vi "Read configuration.vi"(7 "force loading?":bool=TRUE, 8 "error in (no error)":errorcluster, 11 "Galvo in":refnum<class "ImagingModeSPIM.lvclass">) -> (0 "error out":errorcluster, 3 "Galvo out":refnum<class "ImagingModeSPIM.lvclass">)   [LabVIEW 2012, in "ImagingModeSPIM.lvclass"]
doc: "Reads the XML-based configuration file and populates the configuration cluster accordingly. Configuration file name is <component ID>.xml."
uses:
  ImagingModeSPIM.lvclass
  <vilib>/Distrio/Murmex/Murmex/Murmex.lvclass
  ImagingModeSPIM.lvclass/ImagingModeSPIM.ctl
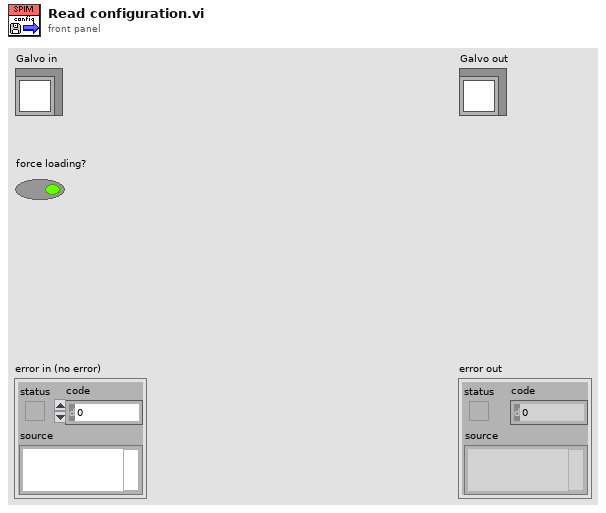
[diagram p1: front panel]
types:
  T1 = typedef "ImagingModeSPIM.lvclass/configuration_cluster.ctl" = cluster{"Sampling rate":dbl, "Samples per channel":i32, "Number of channels":T2, "Task cluster":T3}
  T2 = typedef "ImagingModeSPIM.lvclass/number of channels.ctl" = enum16{"empty", "double sided + PC", "double sided + WFS"}
  T3 = typedef "ImagingModeSPIM.lvclass/task_cluster.ctl" = cluster{"min Voltage":dbl[unit], "max Voltage":dbl[unit], "physical channel":string}
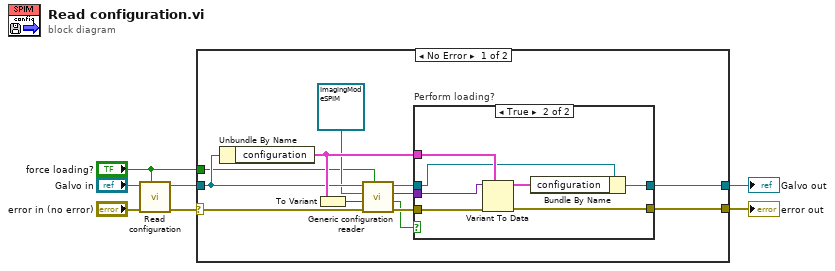
[diagram p0: block diagram]
diagram:
  n1 = call-parent "Read configuration.vi"("force loading?"="force loading?", "error in (no error)"="error in (no error)", "Murmex in"="Galvo in") -> ("error out"=w5:errorcluster, "Murmex out"=w4:refnum<class "ImagingModeSPIM.lvclass">)  [unwired: 7 in]
  n2 = case shown="No Error" w5 {
    selector: w5 -> [w15 w29]
    tunnel: w4 -> [w14 w30]
    tunnel: [w18 w29] -> w3
    tunnel: [w17 w30] -> w2
    tunnel: "force loading?" -> [w9 _]
    frame No Error {
      n3 = Unbundle By Name(w14) -> ("configuration"=w19:T1)
      n4 = To Variant(anything=w19) -> (Variant=w16:variant)
      n5 = call <vilib>:"Generic configuration reader.vi"("force loading?"=w9, "error in (no error)"=w15, "configuration cluster variant"=w16, "inheritance level"=refnum<class "ImagingModeSPIM.lvclass"> refnum ("Galvo.lvclass"), "Murmex in"=w14) -> ("error out"=w12:errorcluster, "loaded?"=w8:bool, "configuration data (variant)"=w10:variant, "Murmex out"=w11:refnum<class "ImagingModeSPIM.lvclass">)  [unwired: 3 in]
      n6 = case "Perform loading?" shown="True" w8 {
        tunnel: w19 -> [_ w28]
        tunnel: [w21 w26] -> w18
        tunnel: [w20 w25] -> w17
        tunnel: w12 -> [w21 w22]
        tunnel: w11 -> [w20 w24]
        tunnel: w10 -> [_ w23]
        frame False {
        }
        frame True {
          n7 = Variant To Data(error in=w22, type=w28, Variant=w23) -> (data=w27:T1, error out=w26:errorcluster)
          n8 = Bundle By Name(cluster=w24, "configuration"=w27) -> (w25:refnum<class "ImagingModeSPIM.lvclass">)
        }
      }
    }
    frame Error {
    }
  }
  "error out" <- w3
  "Galvo out" <- w2
